vi "checkfinishstep.vi"(10 "Step":i32, 11 "StepNumber":i32[](array[numeric])) -> (2 "Step":i32, 3 "ok":bool)   [LabVIEW 2019, in "MPC_VirbVision.lvclass"]
uses:
  MPC_VirbVision.lvclass
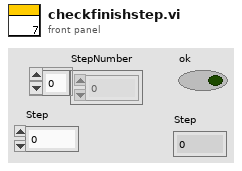
[diagram p1: front panel]
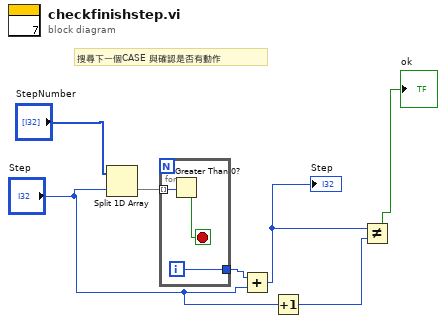
[diagram p0: block diagram]
diagram:
  # "搜尋下一個CASE 與確認是否有動作"
  n1 = Split 1D Array(array="StepNumber", index="Step") -> (second subarray=w6:i32[])  [unwired: 1 out]
  n2 = for {
    tunnel: w6 -> [w10] mode=indexing
    tunnel: [w8] -> w5
    i -> [w8]
    stop <- w9 stop-if-true
    n3 = Greater Than 0?(x=w10) -> (x > 0?=w9:bool)
  }
  n4 = Add(x=w5, y="Step") -> (x+y=w4:i32)
  "Step" <- w4
  n5 = Increment(x="Step") -> (x+1=w2:i32)
  n6 = Not Equal?(x=w4, y=w2) -> (x != y?=→"ok":bool)
